vi "Temperature Acquisition.vi"() -> ()   [LabVIEW 2020]
uses:
  <vilib>/DAQmx/read.llb/DAQmx Read (Analog DBL 1Chan 1Samp).vi
  <vilib>/DAQmx/miscellaneous.llb/DAQmx Fill In Error Info.vi
panel:
  in  "Max Temperature Threshold (deg C)":dbl(slide)=32.91428571428571 scale=15.0..70.0
  out "Message":string
  out "Threshold Exceeded?":bool
  out "Current Temperature (deg C)":dbl
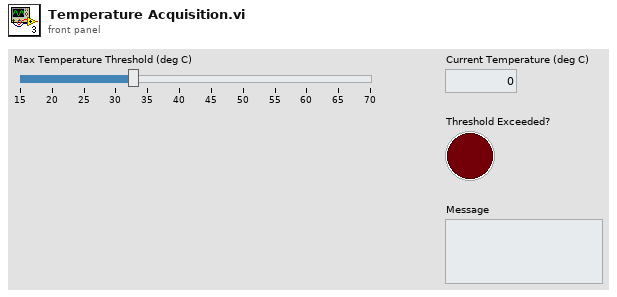
[diagram p1: front panel]
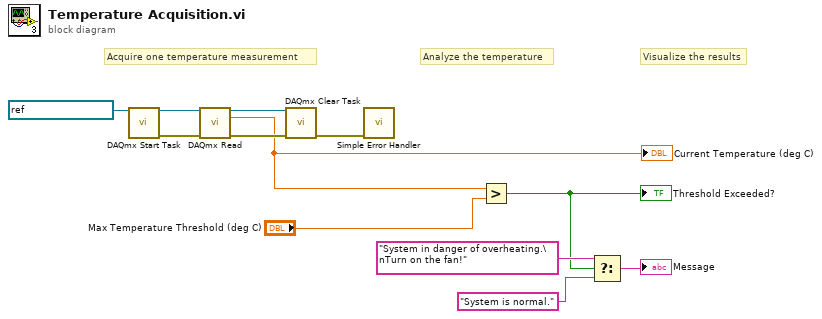
[diagram p0: block diagram]
diagram:
  # "Visualize the results"
  # "Analyze the temperature"
  # "Acquire one temperature measurement"
  n1 = call <vilib>:"DAQmx Start Task.vi"("task/channels in"=refnum<k21> "Thermocouple" ("task in")) -> ("task out"=w12:refnum<k21>, "error out"=w9:errorcluster)  [unwired: 13 in]
  n2 = call-poly <vilib>:"DAQmx Read.vi"("task/channels in"=w12, "error in"=w9) -> ("task out"=w11:refnum<k21>, "data"=w4:dbl, "error out"=w10:errorcluster)  [unwired: 11 in]
  "Current Temperature (deg C)" <- w4
  n3 = call <vilib>:"DAQmx Clear Task.vi"("task in"=w11, "error in"=w10) -> ("error out"=w1:errorcluster)  [unwired: 13 in]
  n4 = call <vilib>:"Simple Error Handler.vi"("error in (no error)"=w1) -> ()  [unwired: 4 in, 5 out]
  n5 = Greater?(x=w4, y="Max Temperature Threshold (deg C)") -> (0:w3:bool)
  "Threshold Exceeded?" <- w3
  n6 = Select(t="System in danger of overheating.\nTurn on the fan!", s=w3, f="System is normal.") -> (s? t:f=→"Message":string)
